vi "is_stable.vi"(4 "milliseconds to wait":u32=100, 5 "max_attempts":i32=100, 6 "sample length":i32=3, 7 "ch":i32=2 min=1 max=4, 8 "error in (no error)":errorcluster, 9 "tolerance":dbl=1e-06 format="%#_6e", 10 "set wavelength (nm)":string="711.4610") -> (0 "error out":errorcluster, 1 "err (nm)":dbl=4.2315184600738576e-07, 2 "rec wavelength (nm)":dbl=711.4610004231519, 3 "attempts":i32)   [LabVIEW 2017, in "highfinesse.lvlib"]
uses:
  highfinesse.lvlib
  wlmData.dll
  <vilib>/ptbypt/NI_PtbyPt.lvlib
panel:
  in  "stop":bool
  out "err":dbl(graph)=4.2315184600738576e-07
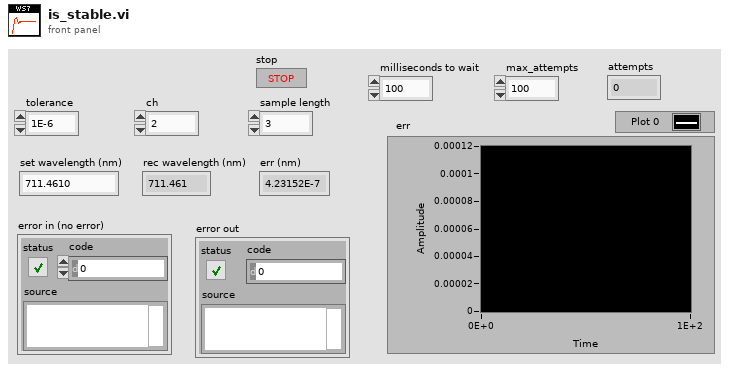
[diagram p1: front panel]
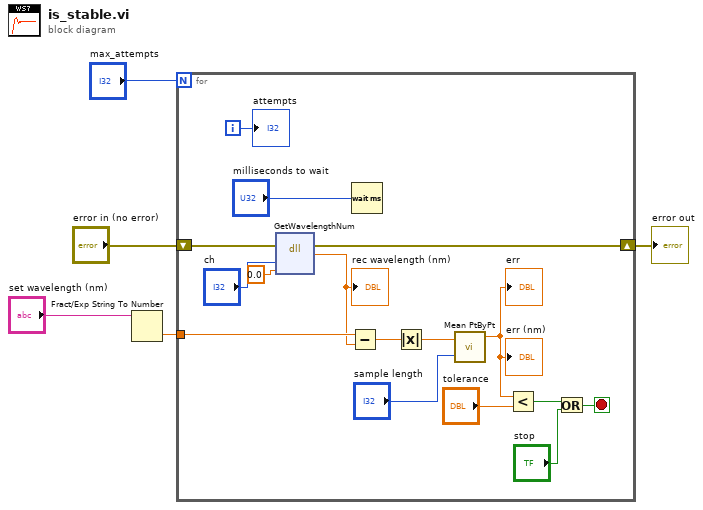
[diagram p0: block diagram]
diagram:
  n1 = Fract/Exp String To Number(string="set wavelength (nm)") -> (number=w4:dbl)  [unwired: 3 in, 1 out]
  n2 = for {
    N: "max_attempts" -> [_]
    tunnel: w4 -> [w21]
    shift-right: [w16] -> w2
    shift-left: "error in (no error)" -> [w17]
    i -> [w6]
    stop <- w7 stop-if-true
    n3 = dll-call lib="wlmData.dll" fn="GetWavelengthNum"(error in=w17, "arg1"="ch", "arg2"=0.0) -> (error out=w16:errorcluster, "return type"=w20:dbl)  [unwired: 4 in, 1 out]
    "rec wavelength (nm)" <- w20
    n4 = Subtract(x=w21, y=w20) -> (x-y=w19:dbl)
    n5 = Wait (ms)(milliseconds to wait="milliseconds to wait") -> ()  [unwired: 1 out]
    n6 = Absolute Value(x=w19) -> (abs(x)=w12:dbl)
    n7 = call <vilib>:"Mean PtByPt.vi"("x"=w12, "sample length"="sample length") -> ("mean"=w11:dbl)  [unwired: 2 in, 1 out]
    "err (nm)" <- w11
    "err" <- w11
    n8 = Less?(x=w11, y="tolerance") -> (x < y?=w9:bool)
    n9 = Or(x=w9, y="stop") -> (x .or. y?=w7:bool)
    "attempts" <- w6
  }
  "error out" <- w2
